vi "Waveform Array to Cluster.vi"(9 "Lengths":i32[](array[numeric]), 10 "Concatenated Waveforms":waveform(dbl)[](array[waveform])) -> (2 "Waveform Cluster":T1)   [LabVIEW 2019, in "Instrument.Lockin.lvlib" / "Instrument.DAQ.lvclass"]
uses:
  Instrument.DAQ.lvclass
  Typedefs/PublicEvents--DAQ.getWaveforms.ctl
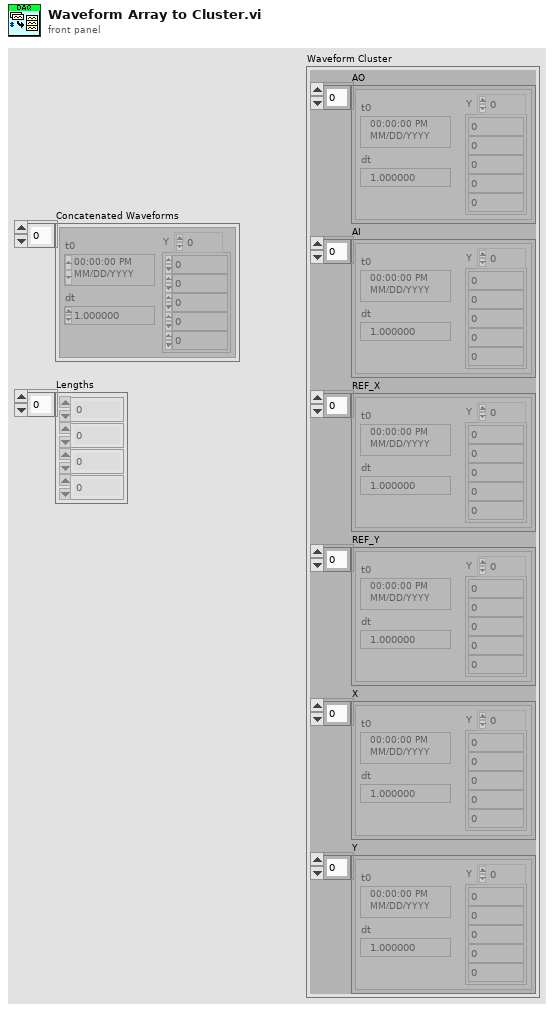
[diagram p1: front panel]
types:
  T1 = typedef "Instrument.Lockin.lvlib/Instrument.DAQ.lvclass/PublicEvents--DAQ.getWaveforms.ctl" = cluster{"AO":waveform(dbl)[], "AI":waveform(dbl)[], "REF_X":waveform(dbl)[], "REF_Y":waveform(dbl)[], "X":waveform(dbl)[], "Y":waveform(dbl)[]}
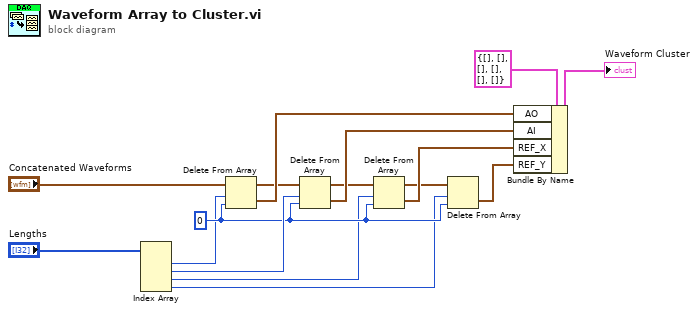
[diagram p0: block diagram]
diagram:
  w9 = 0 ("index")
  n1 = Index Array(array="Lengths") -> (element #1=w8:i32, element #2=w10:i32, element #3=w7:i32, element #4=w6:i32)  [unwired: 4 in]
  n2 = Delete From Array(array="Concatenated Waveforms", length=w8, index=w9) -> (deleted portion=w11:waveform(dbl)[], array with subset deleted=w3:waveform(dbl)[])
  n3 = Delete From Array(array=w3, length=w10, index=w9) -> (deleted portion=w12:waveform(dbl)[], array with subset deleted=w4:waveform(dbl)[])
  n4 = Delete From Array(array=w4, length=w7, index=w9) -> (deleted portion=w13:waveform(dbl)[], array with subset deleted=w5:waveform(dbl)[])
  n5 = Delete From Array(array=w5, length=w6, index=w9) -> (deleted portion=w14:waveform(dbl)[])  [unwired: 1 out]
  n6 = Bundle By Name(cluster=T1 {"AO"=[], "AI"=[], "REF_X"=[], "REF_Y"=[], "X"=[], "Y"=[]} ("Waveforms in"), "AO"=w11, "AI"=w12, "REF_X"=w13, "REF_Y"=w14) -> (→"Waveform Cluster":T1)
